vi "Table Rows Total Time subVI for testing log.vi"(8 "error in (no error)":errorcluster, 11 "Input Matrix":T1) -> (0 "error out":errorcluster, 2 "Total Time (mins)":dbl, 3 "# of Table Rows":dbl)   [LabVIEW 2010]
uses:
  <vilib>/Analysis/Matrix/Datatypes/RealMatrix.ctl
  <vilib>/Analysis/Matrix/NI_Matrix.lvlib
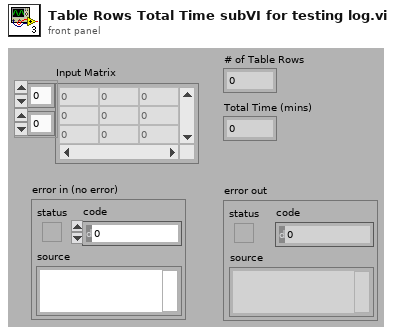
[diagram p1: front panel]
types:
  T1 = typedef "NI_Matrix.lvlib/RealMatrix.ctl" = dbl[][]
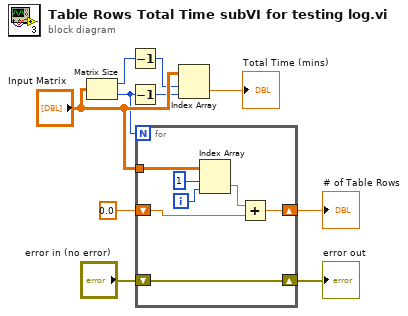
[diagram p0: block diagram]
diagram:
  n1 = Matrix Size(0:"Input Matrix") -> (1:w4:i32, 2:w3:i32)
  n2 = Decrement(x=w4) -> (x-1=w5:i32)
  n3 = Decrement(x=w3) -> (x-1=w2:i32)
  n4 = for {
    N: w3 -> [_]
    shift-right: [w16] -> w9
    shift-left: 0.0 -> [w17]
    tunnel: "Input Matrix" -> [w15]
    shift-right: [w12] -> w7
    shift-left: "error in (no error)" -> [w12]
    i -> [w11]
    n5 = Index Array(array=w15, index (row)=1, index (col)=w11) -> (element=w13:dbl)
    n6 = Add ("Add.vi")(x=w13, y=w17) -> (x+y=w16:dbl)
  }
  "error out" <- w7
  "# of Table Rows" <- w9
  n7 = Index Array(array="Input Matrix", index (row)=w5, index (col)=w2) -> (element=→"Total Time (mins)":dbl)
